vi "report.vi"(0 "Calibration Info":T1, 1 "D":refnum<vi>, 3 "A":refnum<vi>, 5 "Absolute Uncertainties":dbl[](array[numeric]), 7 "data":string[][](array[string]), 8 "H_a":refnum<vi>, 9 "H_d":refnum<vi>, 14 "Equation Asc.":string, 15 "path":path) -> (27 "error out":errorcluster)   [LabVIEW 2021, in "Certification.lvlib"]
uses:
  Certification.lvlib
  <vilib>/Utility/NIReport.llb/Report Type.ctl
  <vilib>/Utility/NIReport.llb/Append Report Text (str wrap).vi
  <vilib>/addons/_office/word.llb/Word Edit Cell ([str]).vi
  <vilib>/ErrorRing/Error Ring.xnode
  <vilib>/Utility/NIReport.llb/NI_report.lvclass
  <vilib>/Utility/NIReport.llb/NI_ReportGenerationCore.lvlib
  <vilib>/addons/_office/NI_ReportGenerationToolkit.lvlib
  <vilib>/Utility/NIReport.llb/Word/NI_Word.lvclass
panel:
  out "exp_abs_uncertainty":dbl
  out "absolute_uncertainty":dbl
  out "mscu":dbl
  out "linearity_error":dbl
  out "hysteresis error":dbl
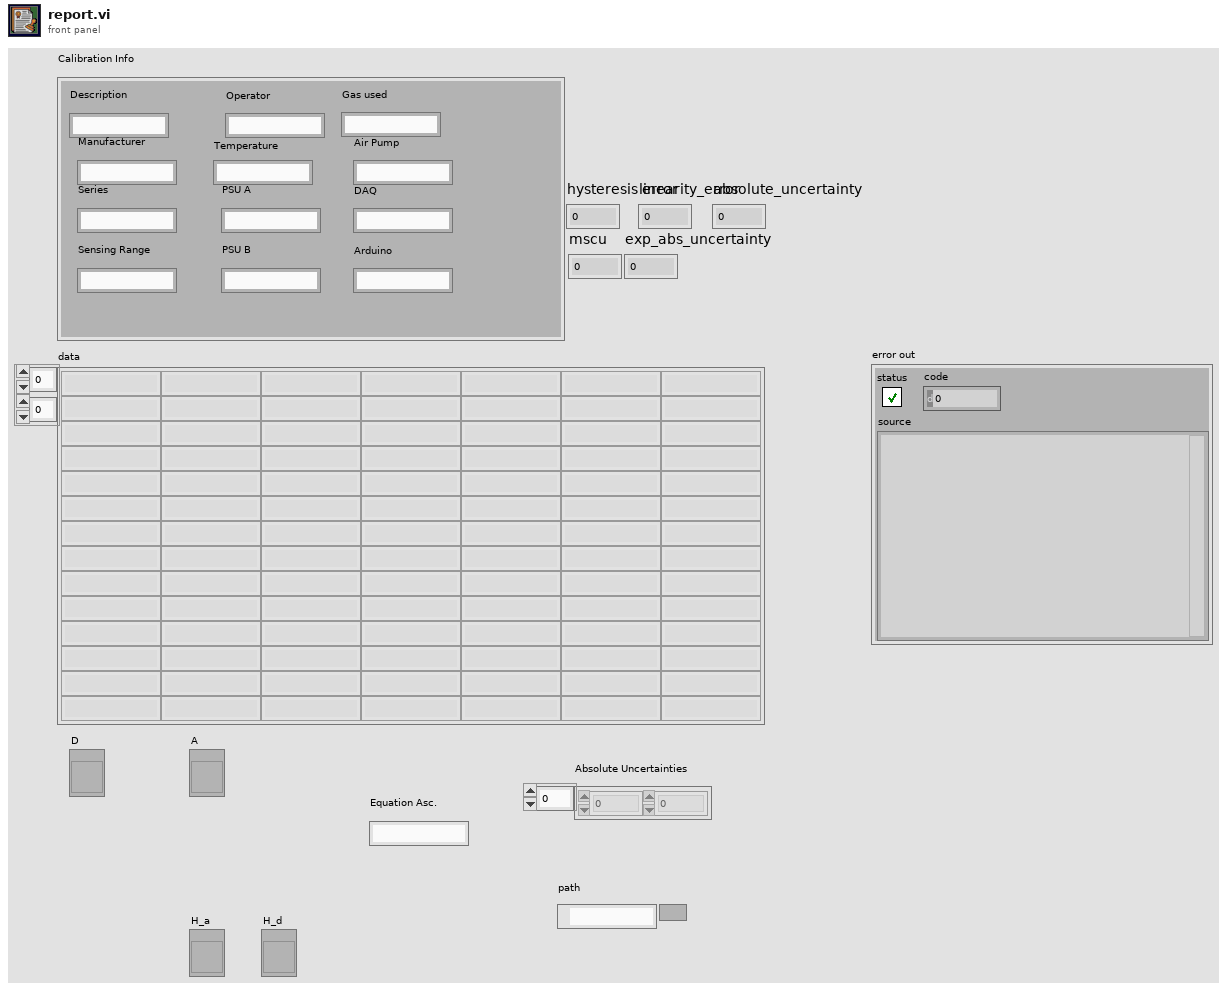
[diagram p1: front panel]
types:
  T1 = cluster{"Description":string, "Manufacturer":string, "Series":string, "Sensing Range":string, "Operator":string, "Temperature":string, "PSU A":string, "PSU B":string, "Gas used":string, "Air Pump":string, "DAQ":string, "Arduino":string}
  T2 = cluster{"position (excel)":cluster{"row":i32, "column":i32}, "name (excel)":string, "bookmark (word)":string}
  T3 = cluster{"position (Excel)":cluster{"row":i32, "column":i32}, "name (Excel)":string, "bookmark (Word)":string}
  T4 = typedef "NI_ReportGenerationCore.lvlib/Report Type.ctl" = enum16{"HTML", "Word", "Excel"}
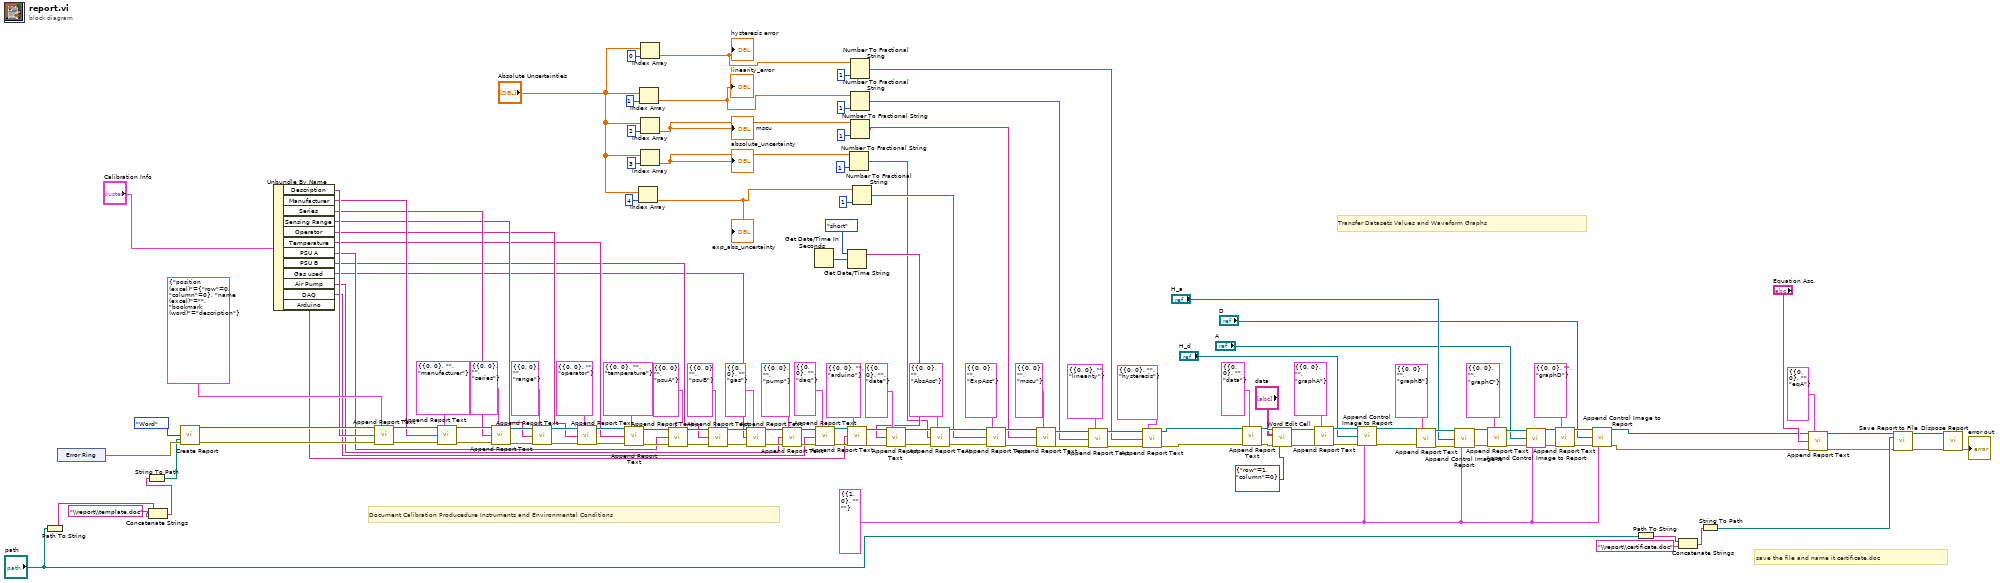
[diagram p0: block diagram]
diagram:
  w7 = T3 {"position (Excel)"={"row"=1, "column"=0}, "name (Excel)"="", "bookmark (Word)"=""} ("MS Office parameters")
  # "save the file and name it certificate.doc"
  # "Transfer Datasets Values and Waveform Graphs"
  # "Document Calibration Producedure Instruments and Environmental Conditions"
  n1 = Path To String(path="path") -> (string=w60:string)
  n2 = xnode "Error Ring"() -> ("error out"=w142:errorcluster)
  n3 = Concatenate Strings(w60, "\\report\\template.doc" ("string")) -> (w62:string)
  n4 = String To Path(string=w62) -> (path=w61:path)
  n5 = call <vilib>:"Create Report.vi"("report type"=Report_Type."Word", "template (empty)"=w61, "error in (no error)"=w142) -> ("report out"=w140:refnum<class "NI_report.lvclass">, "error out"=w141:errorcluster)  [unwired: 11 in]
  n6 = Unbundle By Name("Calibration Info") -> ("Description"=w134:string, "Manufacturer"=w130:string, "Series"=w123:string, "Sensing Range"=w122:string, "Operator"=w118:string, "Temperature"=w114:string, "PSU A"=w110:string, "PSU B"=w106:string, "Gas used"=w103:string, "Air Pump"=w99:string, "DAQ"=w94:string, "Arduino"=w91:string)
  n7 = call-poly <vilib>:"Append Report Text.vi"("report in"=w140, "MS Office parameters"=T2 {"position (excel)"={"row"=0, "column"=0}, "name (excel)"="", "bookmark (word)"="description"}, "text"=w134, "error in (no error)"=w141) -> ("report out"=w133:refnum<class "NI_report.lvclass">, "error out"=w132:errorcluster)  [unwired: 8 in, 2 out]
  n8 = call-poly <vilib>:"Append Report Text.vi"("report in"=w133, "MS Office parameters"=T2 {"position (excel)"={"row"=0, "column"=0}, "name (excel)"="", "bookmark (word)"="manufacturer"}, "text"=w130, "error in (no error)"=w132) -> ("report out"=w129:refnum<class "NI_report.lvclass">, "error out"=w128:errorcluster)  [unwired: 8 in, 2 out]
  n9 = call-poly <vilib>:"Append Report Text.vi"("report in"=w129, "MS Office parameters"=T2 {"position (excel)"={"row"=0, "column"=0}, "name (excel)"="", "bookmark (word)"="series"}, "text"=w123, "error in (no error)"=w128) -> ("report out"=w126:refnum<class "NI_report.lvclass">, "error out"=w125:errorcluster)  [unwired: 8 in, 2 out]
  n10 = call-poly <vilib>:"Append Report Text.vi"("report in"=w126, "MS Office parameters"=T2 {"position (excel)"={"row"=0, "column"=0}, "name (excel)"="", "bookmark (word)"="range"}, "text"=w122, "error in (no error)"=w125) -> ("report out"=w121:refnum<class "NI_report.lvclass">, "error out"=w120:errorcluster)  [unwired: 8 in, 2 out]
  n11 = call-poly <vilib>:"Append Report Text.vi"("report in"=w121, "MS Office parameters"=T2 {"position (excel)"={"row"=0, "column"=0}, "name (excel)"="", "bookmark (word)"="operator"}, "text"=w118, "error in (no error)"=w120) -> ("report out"=w117:refnum<class "NI_report.lvclass">, "error out"=w116:errorcluster)  [unwired: 8 in, 2 out]
  n12 = call-poly <vilib>:"Append Report Text.vi"("report in"=w117, "MS Office parameters"=T2 {"position (excel)"={"row"=0, "column"=0}, "name (excel)"="", "bookmark (word)"="temperature"}, "text"=w114, "error in (no error)"=w116) -> ("report out"=w113:refnum<class "NI_report.lvclass">, "error out"=w112:errorcluster)  [unwired: 8 in, 2 out]
  n13 = Index Array(array="Absolute Uncertainties", index=4) -> (element=w19:dbl)
  "exp_abs_uncertainty" <- w19
  n14 = Index Array(array="Absolute Uncertainties", index=1 ("index (row)")) -> (element=w38:dbl)
  "linearity_error" <- w38
  n15 = Index Array(array="Absolute Uncertainties", index=0 ("index (row)")) -> (element=w43:dbl)
  "hysteresis error" <- w43
  n16 = Index Array(array="Absolute Uncertainties", index=2 ("index (row)")) -> (element=w37:dbl)
  "mscu" <- w37
  n17 = Index Array(array="Absolute Uncertainties", index=3 ("index (row)")) -> (element=w36:dbl)
  "absolute_uncertainty" <- w36
  n18 = call-poly <vilib>:"Append Report Text.vi"("report in"=w113, "MS Office parameters"=T2 {"position (excel)"={"row"=0, "column"=0}, "name (excel)"="", "bookmark (word)"="psuA"}, "text"=w110, "error in (no error)"=w112) -> ("report out"=w109:refnum<class "NI_report.lvclass">, "error out"=w108:errorcluster)  [unwired: 8 in, 2 out]
  n19 = call-poly <vilib>:"Append Report Text.vi"("report in"=w109, "MS Office parameters"=T2 {"position (excel)"={"row"=0, "column"=0}, "name (excel)"="", "bookmark (word)"="psuB"}, "text"=w106, "error in (no error)"=w108) -> ("report out"=w105:refnum<class "NI_report.lvclass">, "error out"=w104:errorcluster)  [unwired: 8 in, 2 out]
  n20 = call-poly <vilib>:"Append Report Text.vi"("report in"=w105, "MS Office parameters"=T2 {"position (excel)"={"row"=0, "column"=0}, "name (excel)"="", "bookmark (word)"="gas"}, "text"=w103, "error in (no error)"=w104) -> ("report out"=w101:refnum<class "NI_report.lvclass">, "error out"=w100:errorcluster)  [unwired: 8 in, 2 out]
  n21 = call-poly <vilib>:"Append Report Text.vi"("report in"=w101, "MS Office parameters"=T2 {"position (excel)"={"row"=0, "column"=0}, "name (excel)"="", "bookmark (word)"="pump"}, "text"=w99, "error in (no error)"=w100) -> ("report out"=w97:refnum<class "NI_report.lvclass">, "error out"=w96:errorcluster)  [unwired: 8 in, 2 out]
  n22 = Get Date/Time In Seconds() -> (seconds since 1Jan1904=w50:timestamp)
  n23 = call-poly <vilib>:"Append Report Text.vi"("report in"=w97, "MS Office parameters"=T2 {"position (excel)"={"row"=0, "column"=0}, "name (excel)"="", "bookmark (word)"="daq"}, "text"=w94, "error in (no error)"=w96) -> ("report out"=w93:refnum<class "NI_report.lvclass">, "error out"=w92:errorcluster)  [unwired: 8 in, 2 out]
  n24 = Get Date/Time String(date format (0)=enum16{"short", "long", "abbreviated"}."short", seconds (now)=w50) -> (date string=w49:string)  [unwired: 1 in, 1 out]
  n25 = call-poly <vilib>:"Append Report Text.vi"("report in"=w93, "MS Office parameters"=T2 {"position (excel)"={"row"=0, "column"=0}, "name (excel)"="", "bookmark (word)"="arduino"}, "text"=w91, "error in (no error)"=w92) -> ("report out"=w53:refnum<class "NI_report.lvclass">, "error out"=w52:errorcluster)  [unwired: 8 in, 2 out]
  n26 = Number To Fractional String(number=w36, precision (6)=i16 1) -> (F-format string=w17:string)  [unwired: 2 in]
  n27 = Number To Fractional String(number=w43, precision (6)=i16 1) -> (F-format string=w12:string)  [unwired: 2 in]
  n28 = Number To Fractional String(number=w38, precision (6)=i16 1) -> (F-format string=w23:string)  [unwired: 2 in]
  n29 = Number To Fractional String(number=w37, precision (6)=i16 1) -> (F-format string=w16:string)  [unwired: 2 in]
  n30 = Number To Fractional String(number=w19, precision (6)=i16 1) -> (F-format string=w18:string)  [unwired: 2 in]
  n31 = call-poly <vilib>:"Append Report Text.vi"("report in"=w53, "MS Office parameters"=T2 {"position (excel)"={"row"=0, "column"=0}, "name (excel)"="", "bookmark (word)"="date"}, "text"=w49, "error in (no error)"=w52) -> ("report out"=w33:refnum<class "NI_report.lvclass">, "error out"=w34:errorcluster)  [unwired: 8 in, 2 out]
  n32 = call-poly <vilib>:"Append Report Text.vi"("report in"=w33, "MS Office parameters"=T2 {"position (excel)"={"row"=0, "column"=0}, "name (excel)"="", "bookmark (word)"="AbsAsc"}, "text"=w17, "error in (no error)"=w34) -> ("report out"=w32:refnum<class "NI_report.lvclass">, "error out"=w31:errorcluster)  [unwired: 8 in, 2 out]
  n33 = call-poly <vilib>:"Append Report Text.vi"("report in"=w32, "MS Office parameters"=T2 {"position (excel)"={"row"=0, "column"=0}, "name (excel)"="", "bookmark (word)"="ExpAsc"}, "text"=w18, "error in (no error)"=w31) -> ("report out"=w29:refnum<class "NI_report.lvclass">, "error out"=w28:errorcluster)  [unwired: 8 in, 2 out]
  n34 = call-poly <vilib>:"Append Report Text.vi"("report in"=w29, "MS Office parameters"=T2 {"position (excel)"={"row"=0, "column"=0}, "name (excel)"="", "bookmark (word)"="mscu"}, "text"=w16, "error in (no error)"=w28) -> ("report out"=w26:refnum<class "NI_report.lvclass">, "error out"=w25:errorcluster)  [unwired: 8 in, 2 out]
  n35 = call-poly <vilib>:"Append Report Text.vi"("report in"=w26, "MS Office parameters"=T2 {"position (excel)"={"row"=0, "column"=0}, "name (excel)"="", "bookmark (word)"="linearity"}, "text"=w23, "error in (no error)"=w25) -> ("report out"=w15:refnum<class "NI_report.lvclass">, "error out"=w14:errorcluster)  [unwired: 8 in, 2 out]
  n36 = call-poly <vilib>:"Append Report Text.vi"("report in"=w15, "MS Office parameters"=T2 {"position (excel)"={"row"=0, "column"=0}, "name (excel)"="", "bookmark (word)"="hysteresis"}, "text"=w12, "error in (no error)"=w14) -> ("report out"=w11:refnum<class "NI_report.lvclass">, "error out"=w10:errorcluster)  [unwired: 8 in, 2 out]
  n37 = call-poly <vilib>:"Append Report Text.vi"("report in"=w11, "MS Office parameters"=T2 {"position (excel)"={"row"=0, "column"=0}, "name (excel)"="", "bookmark (word)"="data"}, "error in (no error)"=w10) -> ("report out"=w82:refnum<class "NI_report.lvclass">, "error out"=w83:errorcluster)  [unwired: 9 in, 2 out]
  n38 = call-poly <vilib>:"Word Edit Cell.vi"("report in"=w82, "value"="data", "error in (no error)"=w83, "start (0, 0)"=cluster{"row":i32, "column":i32} {"row"=1, "column"=0}) -> ("report out"=w85:refnum<class "NI_report.lvclass">, "error out"=w84:errorcluster)  [unwired: 10 in]
  n39 = call-poly <vilib>:"Append Report Text.vi"("report in"=w85, "MS Office parameters"=T2 {"position (excel)"={"row"=0, "column"=0}, "name (excel)"="", "bookmark (word)"="graphA"}, "error in (no error)"=w84) -> ("report out"=w87:refnum<class "NI_report.lvclass">, "error out"=w86:errorcluster)  [unwired: 9 in, 2 out]
  n40 = call-dynamic "Append Control Image to Report.vi"("report in"=w87, "ctrl reference"="H_d", "error in (no error)"=w86, "MS Office parameters"=w7) -> ("report out"=w79:refnum<class "NI_report.lvclass">, "error out"=w78:errorcluster)  [unwired: 8 in, 2 out]
  n41 = call-poly <vilib>:"Append Report Text.vi"("report in"=w79, "MS Office parameters"=T2 {"position (excel)"={"row"=0, "column"=0}, "name (excel)"="", "bookmark (word)"="graphB"}, "error in (no error)"=w78) -> ("report out"=w76:refnum<class "NI_report.lvclass">, "error out"=w75:errorcluster)  [unwired: 9 in, 2 out]
  n42 = call-dynamic "Append Control Image to Report.vi"("report in"=w76, "ctrl reference"="H_a", "error in (no error)"=w75, "MS Office parameters"=w7) -> ("report out"=w71:refnum<class "NI_report.lvclass">, "error out"=w70:errorcluster)  [unwired: 8 in, 2 out]
  n43 = call-poly <vilib>:"Append Report Text.vi"("report in"=w71, "MS Office parameters"=T2 {"position (excel)"={"row"=0, "column"=0}, "name (excel)"="", "bookmark (word)"="graphC"}, "error in (no error)"=w70) -> ("report out"=w72:refnum<class "NI_report.lvclass">, "error out"=w69:errorcluster)  [unwired: 9 in, 2 out]
  n44 = call-dynamic "Append Control Image to Report.vi"("report in"=w72, "ctrl reference"="A", "error in (no error)"=w69, "MS Office parameters"=w7) -> ("report out"=w73:refnum<class "NI_report.lvclass">, "error out"=w68:errorcluster)  [unwired: 8 in, 2 out]
  n45 = call-poly <vilib>:"Append Report Text.vi"("report in"=w73, "MS Office parameters"=T2 {"position (excel)"={"row"=0, "column"=0}, "name (excel)"="", "bookmark (word)"="graphD"}, "error in (no error)"=w68) -> ("report out"=w74:refnum<class "NI_report.lvclass">, "error out"=w67:errorcluster)  [unwired: 9 in, 2 out]
  n46 = call-dynamic "Append Control Image to Report.vi"("report in"=w74, "ctrl reference"="D", "error in (no error)"=w67, "MS Office parameters"=w7) -> ("report out"=w4:refnum<class "NI_report.lvclass">, "error out"=w3:errorcluster)  [unwired: 8 in, 2 out]
  n47 = Path To String(path="path") -> (string=w57:string)
  n48 = Concatenate Strings(w57, "\\report\\certificate.doc" ("string")) -> (w55:string)
  n49 = String To Path(string=w55) -> (path=w54:path)
  n50 = call-poly <vilib>:"Append Report Text.vi"("report in"=w4, "MS Office parameters"=T2 {"position (excel)"={"row"=0, "column"=0}, "name (excel)"="", "bookmark (word)"="eqA"}, "text"="Equation Asc.", "error in (no error)"=w3) -> ("report out"=w2:refnum<class "NI_report.lvclass">, "error out"=w1:errorcluster)  [unwired: 8 in, 2 out]
  n51 = call-dynamic "Save Report to File.vi"("report in"=w2, "report file path"=w54, "error in (no error)"=w1) -> ("report out"=w138:refnum<class "NI_report.lvclass">, "error out"=w137:errorcluster)  [unwired: 11 in]
  n52 = call-dynamic "Dispose Report.vi"("report in"=w138, "error in (no error)"=w137) -> ("error out"=→"error out":errorcluster)  [unwired: 13 in]
